vi "Lockin.DAQ.Configure Sweep 4.vi"(8 "error in (no error)":errorcluster, 11 "Lockin.DAQ in":refnum<class "Lockin.DAQ.lvclass">) -> (0 "error out":errorcluster, 3 "Lockin.DAQ out":refnum<class "Lockin.DAQ.lvclass">)   [LabVIEW 2016, in "Lockin.DAQ.lvclass"]
uses:
  Lockin.DAQ.lvclass
  Lockin.DAQ.lvclass/Lockin.DAQ.ctl
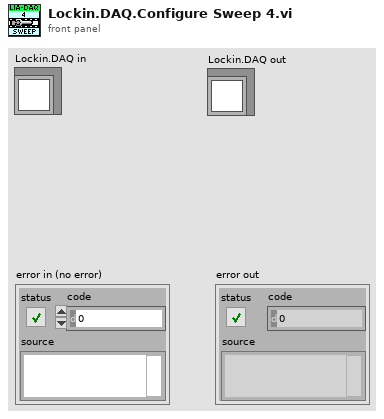
[diagram p1: front panel]
types:
  T1 = typedef "Lockin.DAQ.lvclass/AO-cluster.ctl" = cluster{"Ch":i32[], "Amp (V)":dbl[], "DC (V)":dbl[], "f (Hz)":dbl[], "Phase (°)":dbl[], "Function":T2[], "Sweep?":bool[]}
  T2 = typedef "Lockin.DAQ.lvclass/Function-enum.ctl" = enum16{"Sine", "Triangle", "Square", "Sawtooth"}
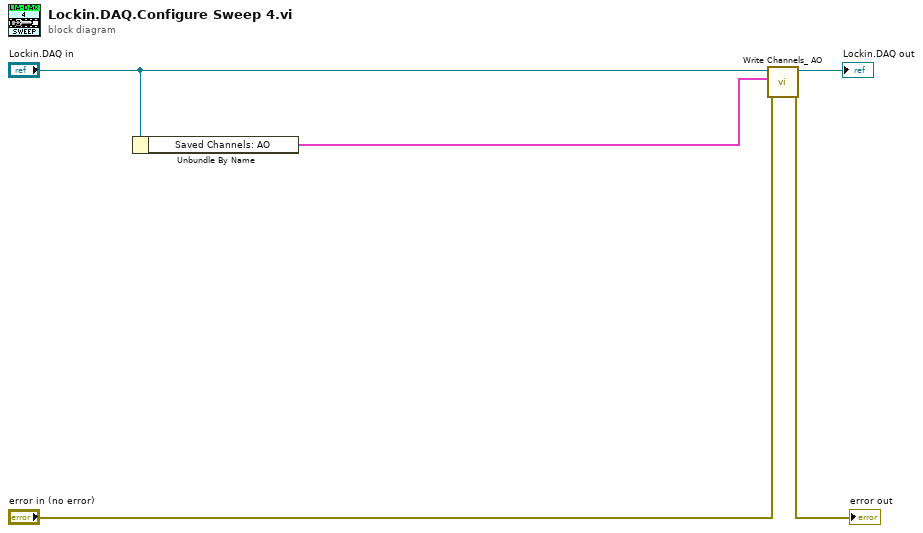
[diagram p0: block diagram]
diagram:
  n1 = Unbundle By Name("Lockin.DAQ in") -> ("Saved Channels: AO"=w1:T1)
  n2 = call "Write Channels_ AO.vi"("error in (no error)"="error in (no error)", "Channels: AO"=w1, "Lockin.DAQ"="Lockin.DAQ in") -> ("error out"=→"error out":errorcluster, "Lockin.DAQ out"=→"Lockin.DAQ out":refnum<class "Lockin.DAQ.lvclass">)  [unwired: 7 in]
